vi "Read SFTP.vi"(8 "Error In":errorcluster, 11 "SFTP File In":refnum<class "SFTP File.lvclass">) -> (0 "Error Out":errorcluster, 2 "SFTP":refnum<class "SFTP.lvclass">, 3 "SFTP File Out":refnum<class "SFTP File.lvclass">)   [LabVIEW 2018, in "Toolkit.lvlib" / "SFTP File.lvclass"]
uses:
  SFTP File.lvclass
  SFTP/SFTP.lvclass
  SFTP File.lvclass/SFTP File.ctl
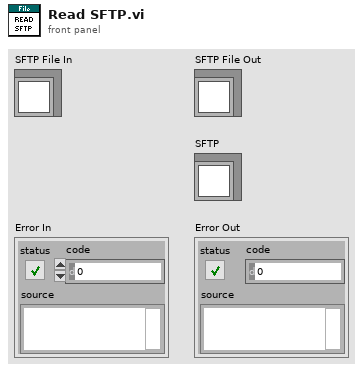
[diagram p1: front panel]
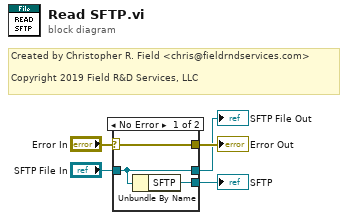
[diagram p0: block diagram]
diagram:
  # "Created by Christopher R. Field <chris@fieldrndservices.com>\n\nCopyright 2019 Field R&D Services, LLC"
  n1 = case shown="No Error" "Error In" {
    selector: "Error In" -> [w8 w10]
    tunnel: "SFTP File In" -> [w7 w9]
    tunnel: [w7 w9] -> w1
    tunnel: [w8 w10] -> w4
    tunnel: [w6 _] -> w3
    frame No Error {
      n2 = Unbundle By Name(w7) -> ("SFTP"=w6:refnum<class "SFTP.lvclass">)
    }
    frame Error {
    }
  }
  "Error Out" <- w4
  "SFTP" <- w3
  "SFTP File Out" <- w1
